vi "LabU_exemplo.vi"() -> ()   [LabVIEW 2015]
panel:
  in  "stop":bool
  in  "Tab Control":T1(tab)
  in  "Setup":bool
  out "Setup OK?":bool
  in  "Function 2":string(combo)="pinMode 02 OUTPUT"
  out "DigOut OK?":bool
  in  "Função 3":string(combo)="digitalWrite 02 HIGH"
  in  "DigOut":bool
  in  "Slide":i32(slide) min=0 max=255 step=1 scale=0.0..255.0
  out "PWMOut OK?":bool
  in  "PWMOut":bool
  in  "Function":string(combo)="analogWrite 03"
  out "Chart":i32(graph)
  in  "Function 3":string(combo)="analogRead A0"
  out "AnalogR OK?":bool
  in  "AnaloGRead":bool
  in  "Function 4":string(combo)="analogWrite 03"
  out "DigitalIn 2":bool
  in  "DigitalIn":bool
  out "result":string
  out "x = y?":bool
  in  "VISA resource name":refnum<visa-resource-name>="COM11"
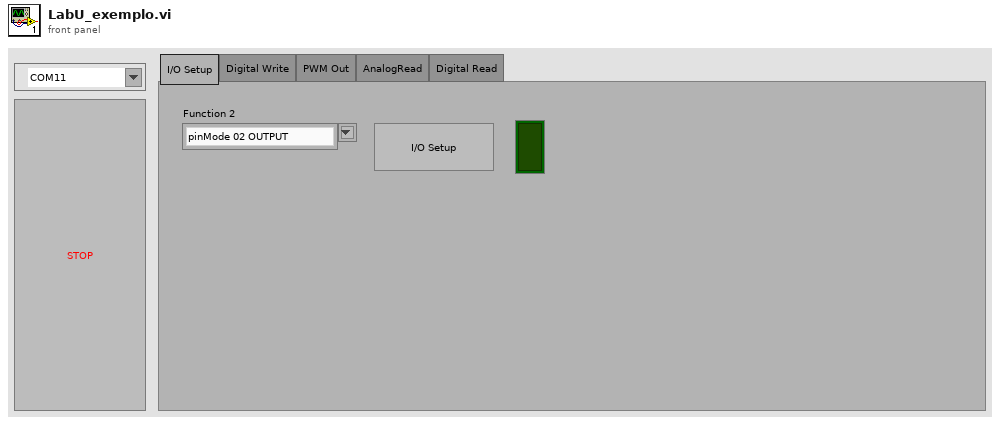
[diagram p1: front panel]
types:
  T1 = enum32{"I/O Setup", "Digital Write", "PWM Out", "AnalogRead", "Digital Read"}
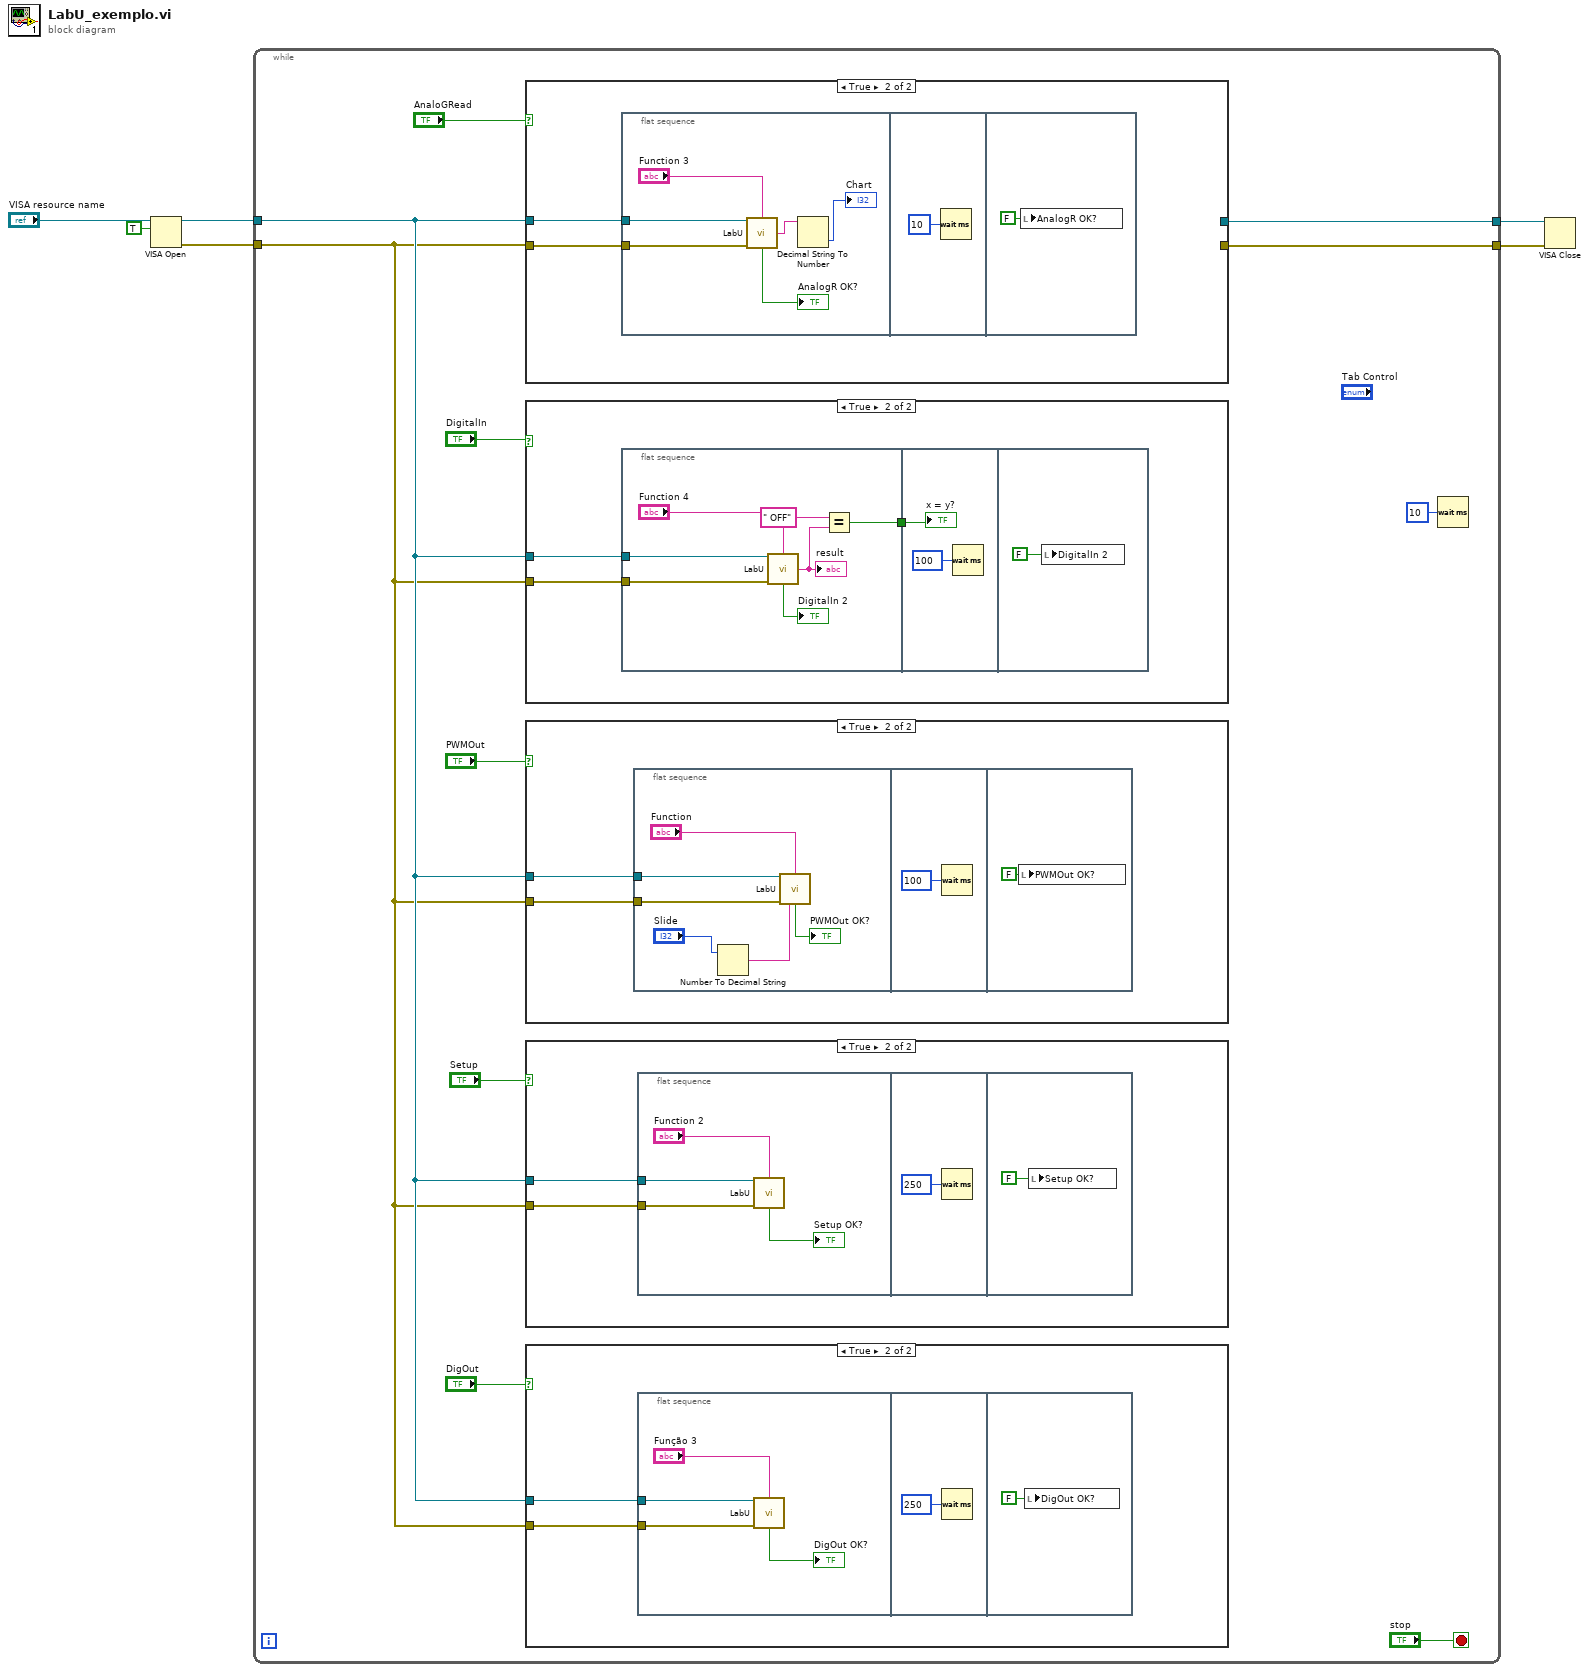
[diagram p0: block diagram]
diagram:
  n1 = VISA Open(duplicate session (F)=TRUE, VISA resource name="VISA resource name") -> (VISA resource name=w3:refnum<visa-resource-name>, error out=w2:errorcluster)  [unwired: 3 in]
  n2 = while {
    tunnel: w3 -> [w9]
    tunnel: [w11] -> w6
    tunnel: w2 -> [w8]
    tunnel: [w10] -> w1
    stop <- "stop" stop-if-true
    n3 = case shown="True" "AnaloGRead" {
      tunnel: w9 -> [w19 w21]
      tunnel: w8 -> [w18 w20]
      tunnel: [w19 _] -> w11
      tunnel: [w18 _] -> w10
      frame False {
      }
      frame True {
        n4 = flat-sequence {
          tunnel: w21 -> [w23]
          tunnel: w20 -> [w22]
          frame #0 {
            n5 = call "LabU.vi"("Serial Com"=w23, "Function"="Function 3", "error in (no error)"=w22) -> ("result"=w25:string, "ok?"=→"AnalogR OK?":bool)  [unwired: 9 in, 2 out]
            n6 = Decimal String To Number(string=w25) -> (number=→"Chart":i32)  [unwired: 2 in, 1 out]
          }
          frame #1 {
            n7 = Wait (ms)(milliseconds to wait=u32 10) -> ()  [unwired: 1 out]
          }
          frame #2 {
            n8 = local write "AnalogR OK?"(FALSE ("ok?")) -> ()
          }
        }
      }
    }
    n9 = case shown="True" "DigitalIn" {
      tunnel: w9 -> [_ w31]
      tunnel: w8 -> [_ w30]
      frame False {
      }
      frame True {
        n10 = flat-sequence {
          tunnel: [w35] -> w32
          tunnel: w31 -> [w34]
          tunnel: w30 -> [w33]
          tunnel: w32 -> [w40]
          frame #0 {
            n11 = call "LabU.vi"("Serial Com"=w34, "Function"="Function 4", "error in (no error)"=w33) -> ("result"=w37:string, "ok?"=→"DigitalIn 2":bool)  [unwired: 9 in, 2 out]
            "result" <- w37
            n12 = Equal?(x=" OFF", y=w37) -> (x = y?=w35:bool)
          }
          frame #1 {
            n13 = Wait (ms)(milliseconds to wait=u32 100) -> ()  [unwired: 1 out]
            "x = y?" <- w40
          }
          frame #2 {
            n14 = local write "DigitalIn 2"(FALSE ("ok?")) -> ()
          }
        }
      }
    }
    n15 = case shown="True" "PWMOut" {
      tunnel: w9 -> [_ w44]
      tunnel: w8 -> [_ w43]
      frame False {
      }
      frame True {
        n16 = flat-sequence {
          tunnel: w44 -> [w48]
          tunnel: w43 -> [w47]
          frame #0 {
            n17 = Number To Decimal String(number="Slide") -> (decimal integer string=w46:string)  [unwired: 1 in]
            n18 = call "LabU.vi"("Serial Com"=w48, "Function"="Function", "error in (no error)"=w47, "Data(PWM)"=w46) -> ("ok?"=→"PWMOut OK?":bool)  [unwired: 8 in, 3 out]
          }
          frame #1 {
            n19 = Wait (ms)(milliseconds to wait=u32 100) -> ()  [unwired: 1 out]
          }
          frame #2 {
            n20 = local write "PWMOut OK?"(FALSE ("ok?")) -> ()
          }
        }
      }
    }
    n21 = case shown="True" "Setup" {
      tunnel: w9 -> [_ w62]
      tunnel: w8 -> [_ w61]
      frame False {
      }
      frame True {
        n22 = flat-sequence {
          tunnel: w62 -> [w64]
          tunnel: w61 -> [w63]
          frame #0 {
            n23 = call "LabU.vi"("Serial Com"=w64, "Function"="Function 2", "error in (no error)"=w63) -> ("ok?"=→"Setup OK?":bool)  [unwired: 9 in, 3 out]
          }
          frame #1 {
            n24 = Wait (ms)(milliseconds to wait=u32 250) -> ()  [unwired: 1 out]
          }
          frame #2 {
            n25 = local write "Setup OK?"(FALSE ("ok?")) -> ()
          }
        }
      }
    }
    n26 = case shown="True" "DigOut" {
      tunnel: w9 -> [_ w54]
      tunnel: w8 -> [_ w53]
      frame False {
      }
      frame True {
        n27 = flat-sequence {
          tunnel: w54 -> [w56]
          tunnel: w53 -> [w55]
          frame #0 {
            n28 = call "LabU.vi"("Serial Com"=w56, "Function"="Função 3", "error in (no error)"=w55) -> ("ok?"=→"DigOut OK?":bool)  [unwired: 9 in, 3 out]
          }
          frame #1 {
            n29 = Wait (ms)(milliseconds to wait=u32 250) -> ()  [unwired: 1 out]
          }
          frame #2 {
            n30 = local write "DigOut OK?"(FALSE ("ok?")) -> ()
          }
        }
      }
    }
    n31 = Wait (ms)(milliseconds to wait=u32 10) -> ()  [unwired: 1 out]
  }
  n32 = VISA Close(VISA resource name=w6, error in (no error)=w1) -> ()  [unwired: 1 out]
